vi "CreateMeasureNode.vi"(7 "DOM Document":refnum<k20>, 8 "Error In":errorcluster, 11 "Measure Configuration":T1={"Enabled?"=FALSE, "Count"=1, "Interval (sec)"=0.025, "Voltage Auto Range Enabled?"=TRUE, "Voltage High Limit (V or A)"=0.0, "Voltage Low Limit (V or A)"=0.0, "Current Auto Range Enabled?"=TRUE, "Current High Limit (V or A)"=0.0, "Current Low Limit (V or A)"=0.0} {"Count" min=1 step=1}) -> (0 "Error Out":errorcluster, 3 "Measure Node":refnum<k20>)   [LabVIEW 2013]
uses:
  MeasureConfiguration.ctl
  libs/LV-Utilities/LV-Utilities.lvlib
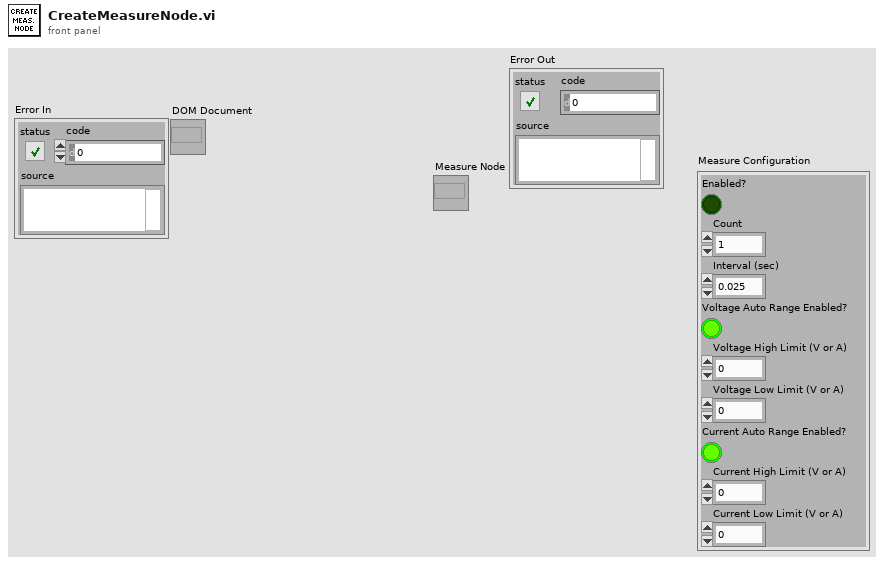
[diagram p1: front panel]
types:
  T1 = typedef "MeasureConfiguration.ctl" = cluster{"Enabled?":bool, "Count":u8, "Interval (sec)":dbl, "Voltage Auto Range Enabled?":bool, "Voltage High Limit (V or A)":dbl, "Voltage Low Limit (V or A)":dbl, "Current Auto Range Enabled?":bool, "Current High Limit (V or A)":dbl, "Current Low Limit (V or A)":dbl}
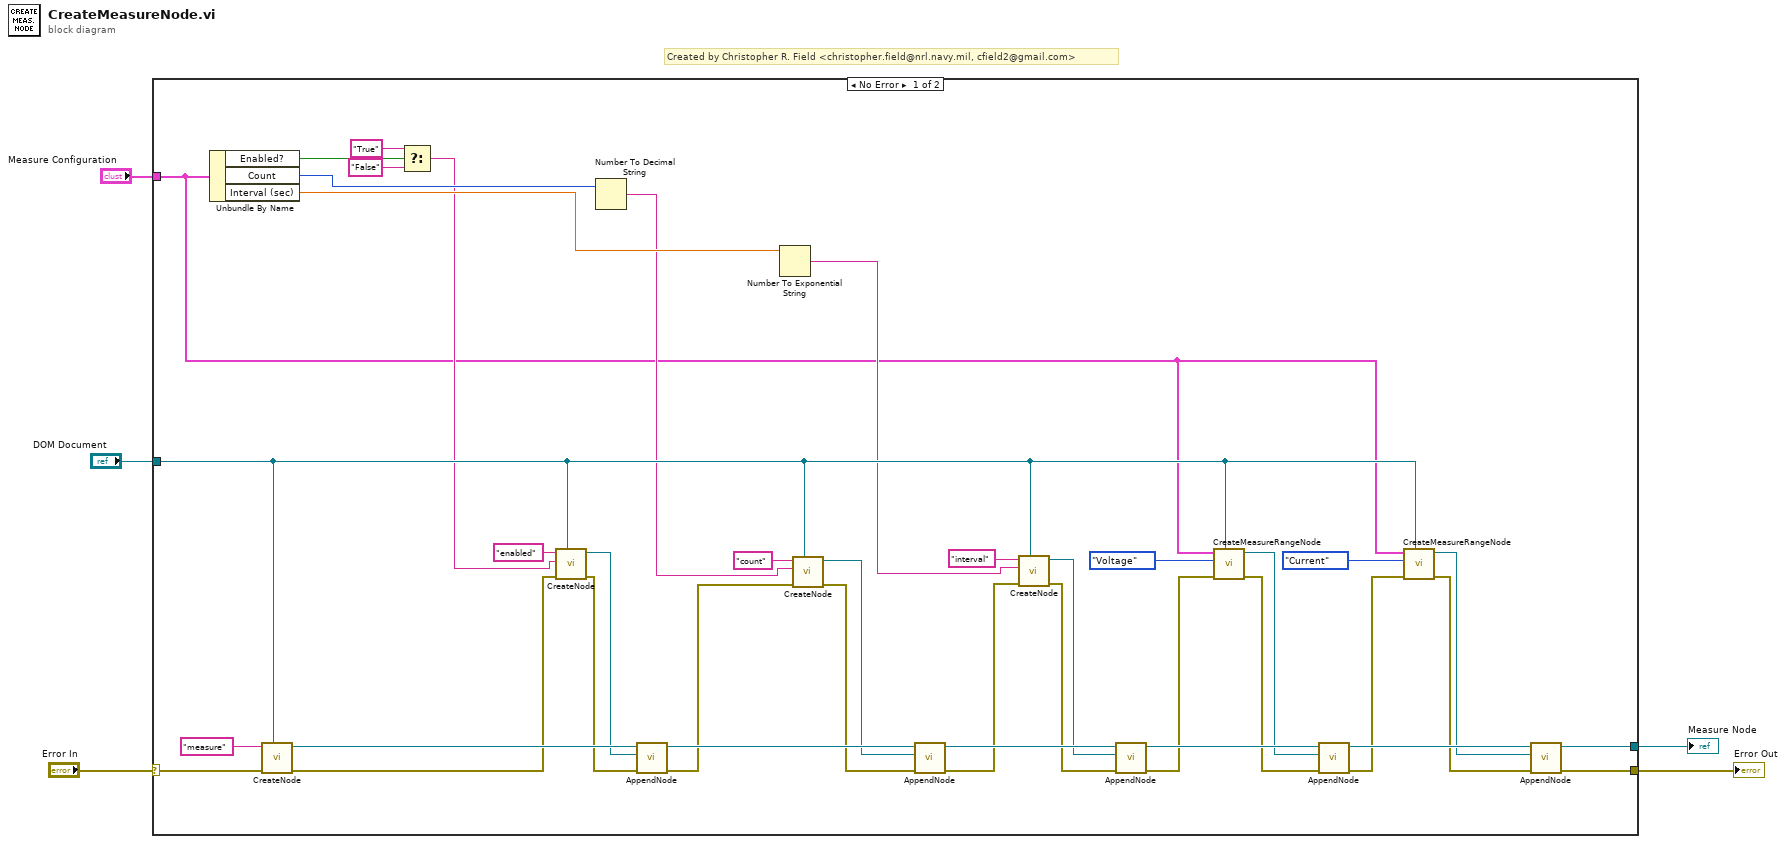
[diagram p0: block diagram]
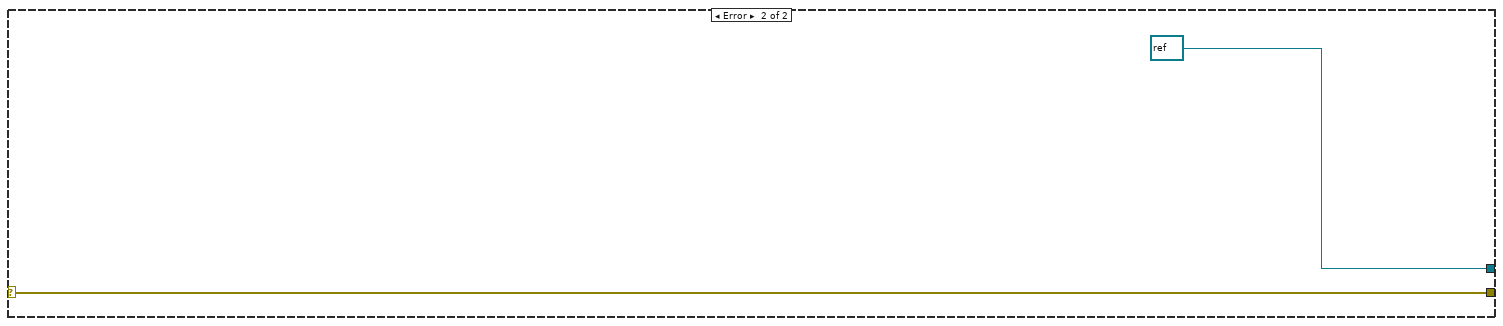
[diagram p2: hidden frame]
diagram:
  # "Created by Christopher R. Field <christopher.field@nrl.navy.mil, cfield2@gmail.com>"
  n1 = case shown="No Error" "Error In" {
    selector: "Error In" -> [w39 w46]
    tunnel: "DOM Document" -> [w12 _]
    tunnel: [w32 refnum<k20> refnum ("Wirings Node 2")] -> w3
    tunnel: [w31 w46] -> w2
    tunnel: "Measure Configuration" -> [w6 _]
    frame No Error {
      n2 = Unbundle By Name(w6) -> ("Enabled?"=w44:bool, "Count"=w40:u8, "Interval (sec)"=w41:dbl)
      n3 = call "CreateNode.vi"("DOM Document"=w12, "Error In"=w39, "Tag Name"="measure") -> ("Error out"=w26:errorcluster, "Node"=w37:refnum<k20>)  [unwired: 7 in]
      n4 = Select(t="True", s=w44, f="False") -> (s? t:f=w7:string)
      n5 = call "CreateNode.vi"("DOM Document"=w12, "Error In"=w26, "Text"=w7, "Tag Name"="enabled") -> ("Error out"=w25:errorcluster, "Node"=w13:refnum<k20>)  [unwired: 6 in]
      n6 = Number To Decimal String(number=w40) -> (decimal integer string=w8:string)  [unwired: 1 in]
      n7 = call "AppendNode.vi"("Error In"=w25, "Child Node"=w13, "Parent Node In"=w37) -> ("Error Out"=w24:errorcluster, "Parent Node Out"=w36:refnum<k20>)  [unwired: 7 in]
      n8 = Number To Exponential String(number=w41) -> (E-format string=w9:string)  [unwired: 3 in]
      n9 = call "CreateNode.vi"("DOM Document"=w12, "Error In"=w24, "Text"=w8, "Tag Name"="count") -> ("Error out"=w23:errorcluster, "Node"=w14:refnum<k20>)  [unwired: 6 in]
      n10 = call "AppendNode.vi"("Error In"=w23, "Child Node"=w14, "Parent Node In"=w36) -> ("Error Out"=w22:errorcluster, "Parent Node Out"=w35:refnum<k20>)  [unwired: 7 in]
      n11 = call "CreateNode.vi"("DOM Document"=w12, "Error In"=w22, "Text"=w9, "Tag Name"="interval" ("Text")) -> ("Error out"=w21:errorcluster, "Node"=w15:refnum<k20>)  [unwired: 6 in]
      n12 = call "AppendNode.vi"("Error In"=w21, "Child Node"=w15, "Parent Node In"=w35) -> ("Error Out"=w20:errorcluster, "Parent Node Out"=w34:refnum<k20>)  [unwired: 7 in]
      n13 = call "CreateMeasureRangeNode.vi"("DOM Document"=w12, "Error In"=w20, "Range Function"=enum16{"Voltage", "Current"}."Voltage", "Measure Configuration"=w6) -> ("Error Out"=w19:errorcluster, "Range Node"=w16:refnum<k20>)  [unwired: 6 in]
      n14 = call "AppendNode.vi"("Error In"=w19, "Child Node"=w16, "Parent Node In"=w34) -> ("Error Out"=w18:errorcluster, "Parent Node Out"=w33:refnum<k20>)  [unwired: 7 in]
      n15 = call "CreateMeasureRangeNode.vi"("DOM Document"=w12, "Error In"=w18, "Range Function"=enum16{"Voltage", "Current"}."Current", "Measure Configuration"=w6) -> ("Error Out"=w30:errorcluster, "Range Node"=w17:refnum<k20>)  [unwired: 6 in]
      n16 = call "AppendNode.vi"("Error In"=w30, "Child Node"=w17, "Parent Node In"=w33) -> ("Error Out"=w31:errorcluster, "Parent Node Out"=w32:refnum<k20>)  [unwired: 7 in]
    }
    frame Error {
    }
  }
  "Measure Node" <- w3
  "Error Out" <- w2
